vi "Read Create Tags_.vi"(8 "error in (no error)":errorcluster, 11 "CVT configuration in":refnum<class "CVT configuration.lvclass">) -> (0 "error out":errorcluster, 2 "Create Tags?":bool=TRUE, 3 "CVT configuration out":refnum<class "CVT configuration.lvclass">)   [LabVIEW 2013, in "CVT configuration.lvclass"]
uses:
  CVT configuration.lvclass
  CVT configuration.lvclass/CVT configuration.ctl
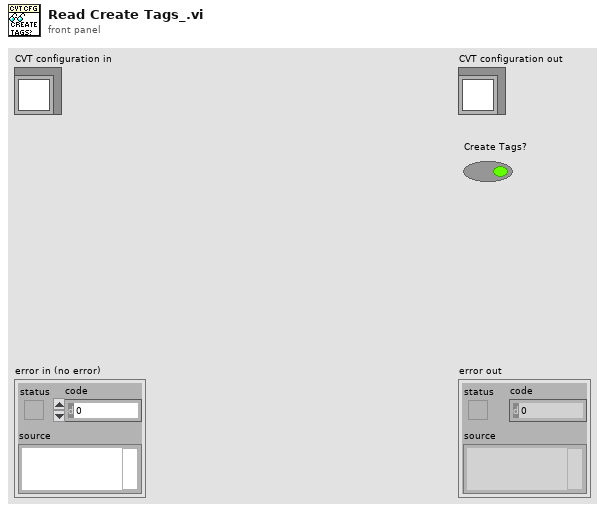
[diagram p1: front panel]
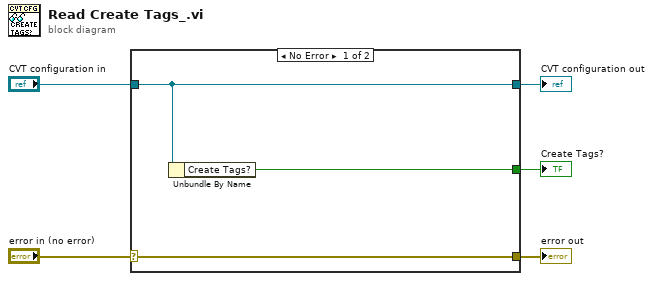
[diagram p0: block diagram]
diagram:
  n1 = case shown="No Error" "error in (no error)" {
    selector: "error in (no error)" -> [w8 w9]
    tunnel: [w8 w9] -> w4
    tunnel: [w7 w10] -> w2
    tunnel: "CVT configuration in" -> [w7 w10]
    tunnel: [w6 _] -> w1
    frame No Error {
      n2 = Unbundle By Name(w7) -> ("Create Tags?"=w6:bool)
    }
    frame Error {
    }
  }
  "error out" <- w4
  "CVT configuration out" <- w2
  "Create Tags?" <- w1
